vi "Measure.vi"(7 "Auto Range (T:Enable)":bool=TRUE, 8 "error in":errorcluster, 9 "Manual Range (1.0)":dbl=1.0, 10 "Function (0: DC Volts)":u16(ring) items=["DC Volts", "AC Volts", "DC Current", "AC Current"], 11 "VISA resource name":refnum<visa-resource-name>) -> (0 "error out":errorcluster, 2 "Measured Value":dbl, 3 "VISA resource name out":refnum<visa-resource-name>)   [LabVIEW 2013, in "DmmPwr Simulator.lvlib"]
uses:
  <instrlib>/DmmPwr Simulator/DmmPwr Simulator.lvlib
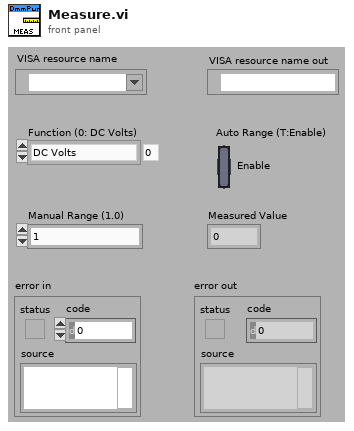
[diagram p1: front panel]
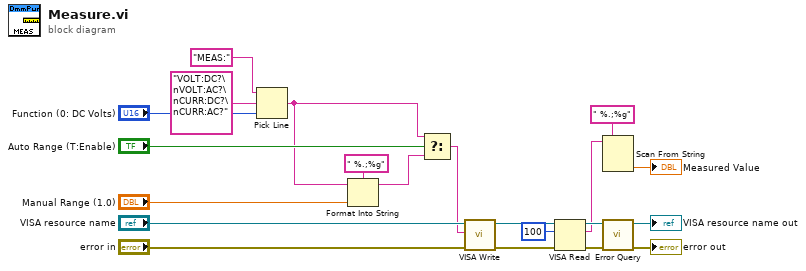
[diagram p0: block diagram]
diagram:
  n1 = Pick Line(string ("")="MEAS:" ("multi-line string"), multi-line string="VOLT:DC?\nVOLT:AC?\nCURR:DC?\nCURR:AC?", line index="Function (0: DC Volts)") -> (output string=w1:string)
  n2 = Format Into String(format string=" %.;%g", initial string=w1, "Manual Range (1.0)") -> (resulting string=w2:string)  [unwired: 1 in, 1 out]
  n3 = Select(t=w1, s="Auto Range (T:Enable)", f=w2) -> (s? t:f=w10:string)
  n4 = call <instrlib>:"VISA Write.vi"("error in"="error in", "write buffer"=w10, "VISA resource name"="VISA resource name") -> ("error out"=w19:errorcluster, "VISA resource name out"=w18:refnum<visa-resource-name>)  [unwired: 6 in, 1 out]
  n5 = VISA Read(VISA resource name=w18, byte count=u32 100, error in (no error)=w19) -> (VISA resource name out=w9:refnum<visa-resource-name>, read buffer=w5:string, error out=w6:errorcluster)  [unwired: 1 out]
  n6 = Scan From String(format string=" %.;%g", input string=w5) -> (output 1=→"Measured Value":dbl)  [unwired: 3 in, 3 out]
  n7 = call <instrlib>:"Error Query.vi"("error in (no error)"=w6, "VISA resource name"=w9) -> ("error out"=→"error out":errorcluster, "VISA resource name out"=→"VISA resource name out":refnum<visa-resource-name>)  [unwired: 6 in, 2 out]
